vi "Filter Noise.vi"(8 "error in":errorcluster caption="error out") -> (0 "error out":errorcluster caption="error in")   [LabVIEW 2015, in "Debug.lvlib"]
uses:
  Debug.lvlib
  Support/Filter Noise State.ctl
  Sub VIs/DAQ/DAQ.lvlib
  Sub VIs/Utility VIs/Utility VIs.lvlib
  Sub VIs/Digital Signal Processing/Digital Signal Processing.lvlib
panel:
  out "进度条":u8(slide) scale=0.0..100.0
  out "DSP":dbl[](graph)
  out "Original Signal":dbl[](graph)
  in  "DOUT":bool
  in  "计算":bool
  in  "采集":bool
  out "状态栏":string
  in  "停止按钮":bool
  # "Filter Noise"
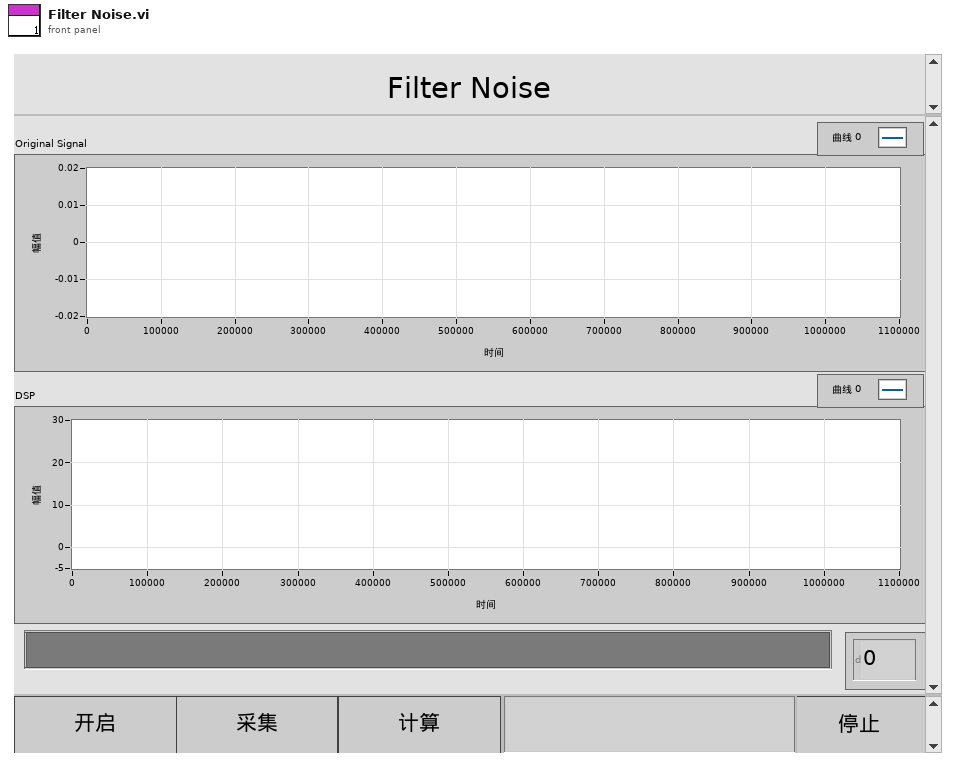
[diagram p1: front panel]
types:
  T1 = typedef "Debug.lvlib/Filter Noise State.ctl" = enum16{"Initialize", "Update Settings", "DOUT", "Sample", "Calculate", "Wait For Event", "Exit"}
  T2 = typedef "DAQ.lvlib/DAQ Configuration.ctl" = cluster{"hDevice":i32, "DevNum":u8, "Configuration Parameter":i32[], "READ_MAX_LEN":i32, "DO":bool[]}
  T3 = typedef "Digital Signal Processing.lvlib/DSP Configuration.ctl" = cluster{"Sampling Frequency":dbl, "filter type":T4, "RF Filter Low Frequency":dbl, "RF Filter High Frequency":dbl, "RF Filter Taps":i32, "window":T5, "RF window parameter":dbl, "filter type 2":T4, "Demodulated Filter Low Frequency":dbl, "Demodulated Filter HighFrequency":dbl, "Demodulated Filter Order":i32, "SPAN":i32, "Logarithmic Base":dbl, "Noise path":string, "Work position parameter":i32[]}
  T4 = typedef "NI_AALBase.lvlib/Filter Passband Type.ctl" = enum32{"Lowpass", "Highpass", "Bandpass", "Bandstop"}
  T5 = typedef "NI_AALPro.lvlib/windowTd.ctl" = u32
  T6 = typedef "Digital Signal Processing.lvlib/DSP Parameter.ctl" = cluster{"RF":cluster{"filter structure":enum32{"IIR 2nd Order", "IIR 4th Order"}, "Reverse Coefficients":dbl[], "Forward Coefficients":dbl[]}, "IIR Filter Cluster":cluster{"filter structure":enum32{"IIR 2nd Order", "IIR 4th Order"}, "Reverse Coefficients":dbl[], "Forward Coefficients":dbl[]}, "Noise Signal":dbl[], "SPAN":i32, "Logarithmic Base":dbl}
  T7 = cluster{"filter structure":enum32{"IIR 2nd Order", "IIR 4th Order"}, "Reverse Coefficients":dbl[], "Forward Coefficients":dbl[]}
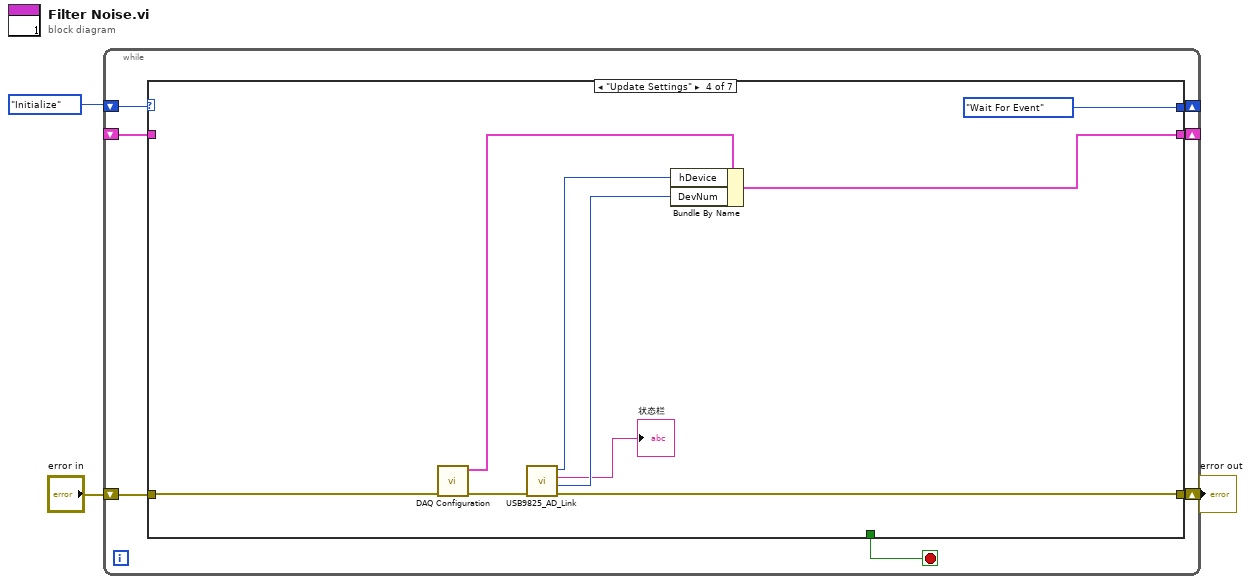
[diagram p0: block diagram]
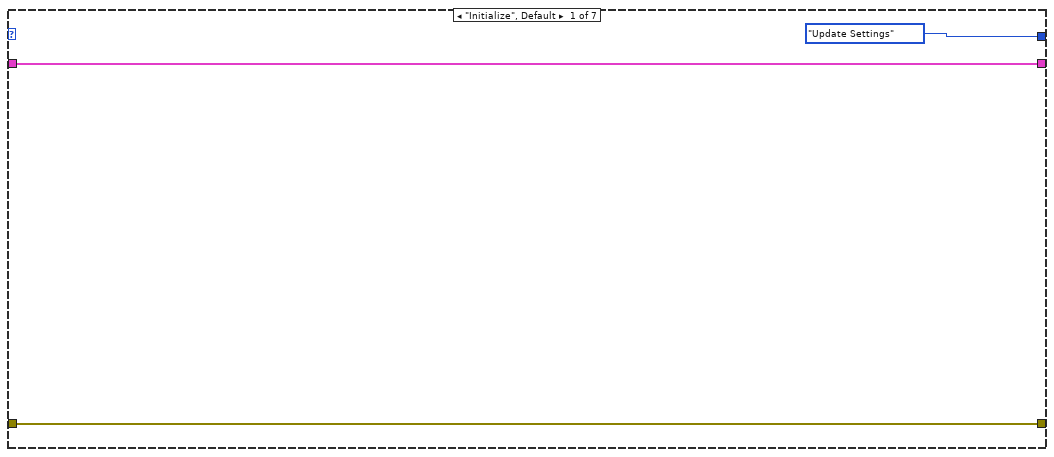
[diagram p2: hidden frame]
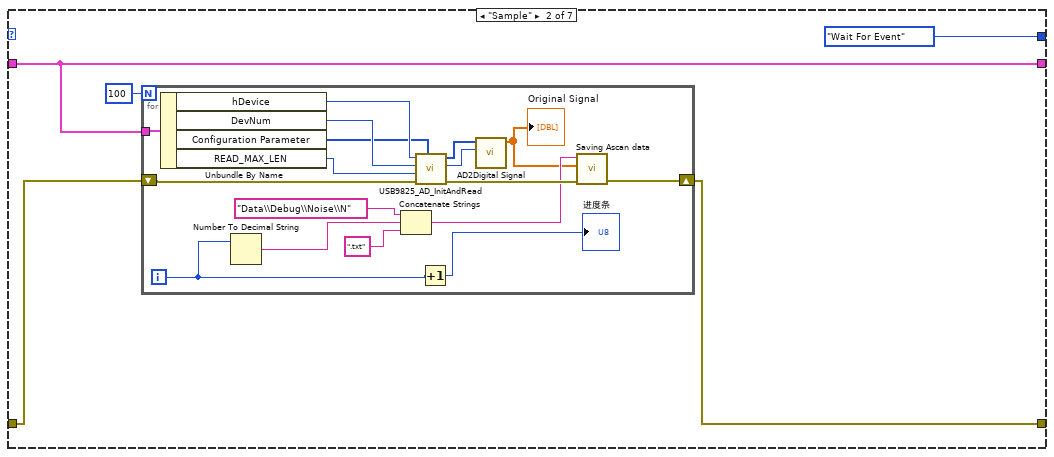
[diagram p3: hidden frame]
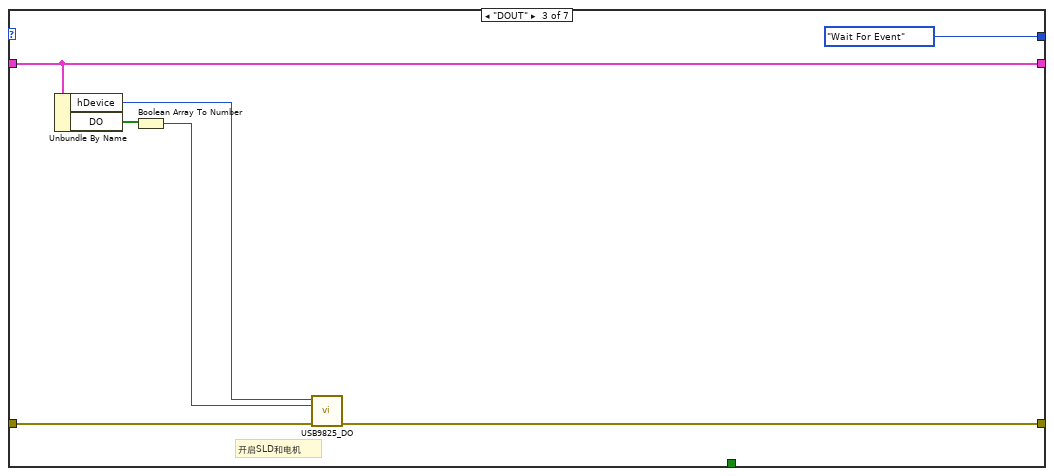
[diagram p4: hidden frame]
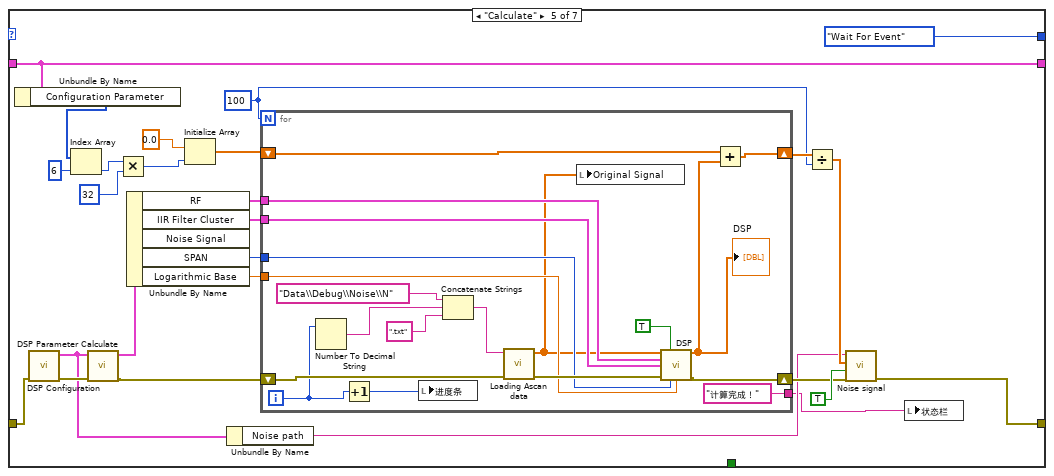
[diagram p5: hidden frame]
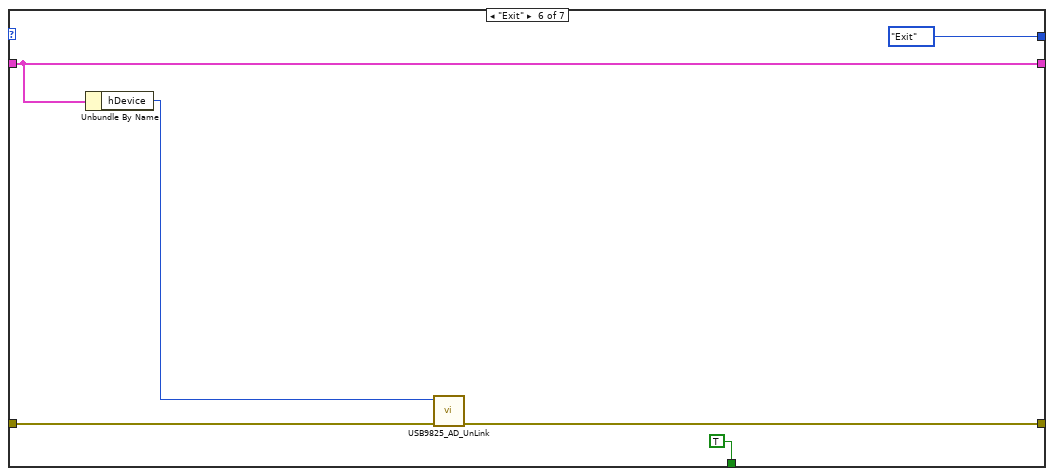
[diagram p6: hidden frame]
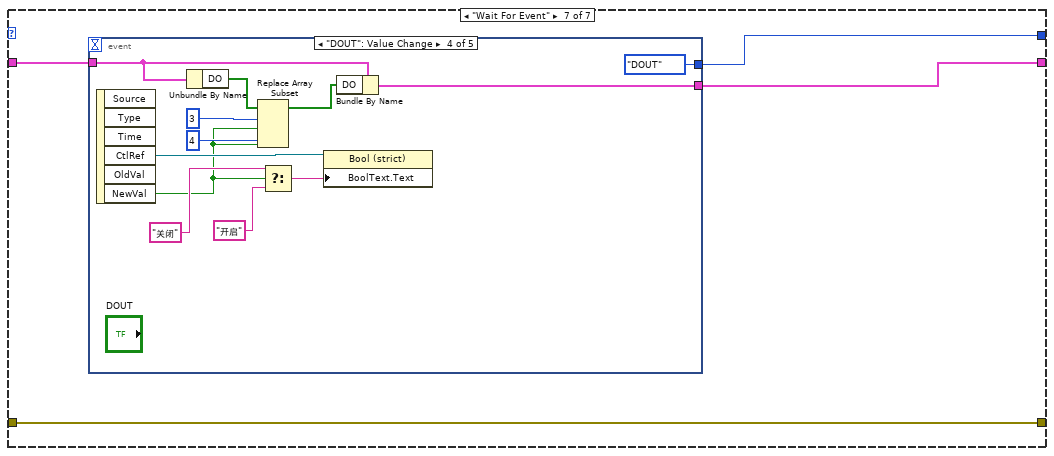
[diagram p7: hidden frame]
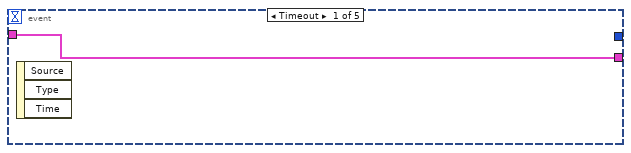
[diagram p8: hidden frame]
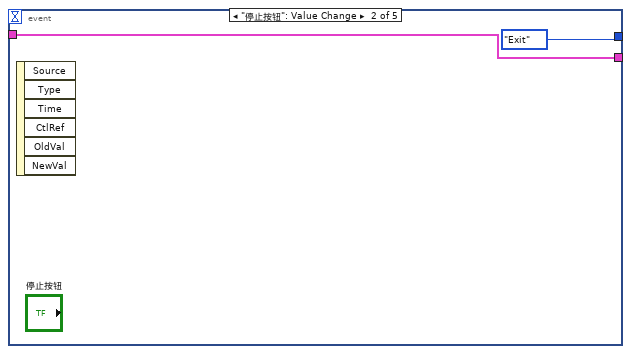
[diagram p9: hidden frame]
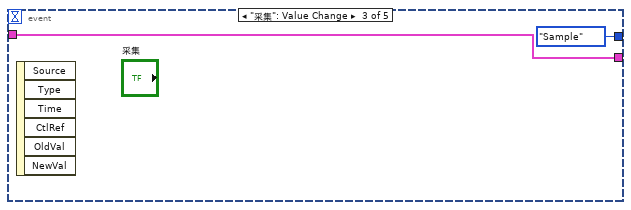
[diagram p10: hidden frame]
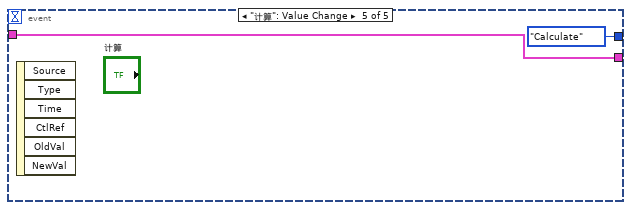
[diagram p11: hidden frame]
diagram:
  n1 = while {
    shift-right: [w9] -> _
    shift-left: Filter_Noise_State."Initialize" ("Calculation Distance State") -> [w10]
    shift-right: [w7] -> w2
    shift-left: "error in" -> [w6]
    shift-right: [w5] -> _
    shift-left: _ -> [w4]
    stop <- w8 stop-if-true
    n2 = case shown="\"Update Settings\"" w10 {
      tunnel: [Filter_Noise_State."Update Settings" ("Calculation Distance State") Filter_Noise_State."Wait For Event" ("Calculation Distance State") Filter_Noise_State."Wait For Event" ("Calculation Distance State") Filter_Noise_State."Wait For Event" ("Calculation Distance State") Filter_Noise_State."Wait For Event" ("Calculation Distance State") Filter_Noise_State."Exit" ("Calculation Distance State") w106] -> w9
      tunnel: [_ _ _ _ _ TRUE _] -> w8
      tunnel: w6 -> [w13 w17 w41 w50 w68 w100 w105]
      tunnel: [w13 w14 w40 w48 w53 w99 w105] -> w7
      tunnel: [w11 w15 w39 w44 w70 w98 w103] -> w5
      tunnel: w4 -> [w11 w15 w39 _ w70 w98 w104]
      frame "Initialize", Default {
      }
      frame "Sample" {
        n3 = for {
          N: 100 -> [_]
          tunnel: w15 -> [w35]
          shift-right: [w28] -> w14
          shift-left: w17 -> [w30]
          i -> [w20]
          n4 = Unbundle By Name(w35) -> ("hDevice"=w34:i32, "DevNum"=w33:u8, "Configuration Parameter"=w31:i32[], "READ_MAX_LEN"=w32:i32)
          n5 = Number To Decimal String(number=w20) -> (decimal integer string=w26:string)  [unwired: 1 in]
          n6 = Concatenate Strings("Data\\Debug\\Noise\\N" ("名称或相对路径"), w26, ".txt" ("字符串")) -> (w24:string)
          n7 = call "USB9825_AD_InitAndRead.vi"("Configuration Parameter"=w31, "错误输入（无错误）"=w30, "READ_MAX_LEN"=w32, "DevNum"=w33, "hDevice"=w34) -> ("错误输出"=w29:errorcluster, "通道数"=w22:i32, "AD"=w23:i16[])  [unwired: 3 in, 1 out]
          n8 = Increment(x=w20) -> (x+1=→"进度条":i32)
          n9 = call "AD2Digital Signal.vi"("通道数"=w22, "AD"=w23) -> ("CH1"=w21:dbl[])  [unwired: 8 in, 1 out]
          "Original Signal" <- w21
          n10 = call "Saving Ascan data.vi"("error in (no error)"=w29, "Ascan Data"=w21, "名称或相对路径"=w24) -> ("error out"=w28:errorcluster)  [unwired: 8 in]
        }
      }
      frame "DOUT" {
        # "开启SLD和电机"
        n11 = Unbundle By Name(w39) -> ("hDevice"=w38:i32, "DO"=w37:bool[])
        n12 = Boolean Array To Number(Boolean array=w37) -> (number=w36:u32)
        n13 = call "USB9825_DO.vi"("Error In"=w41, "pDO"=w36, "hDevice"=w38) -> ("Error Out"=w40:errorcluster)  [unwired: 8 in]
      }
      frame "Update Settings" {
        n14 = call "DAQ Configuration.vi"("error in (no error)"=w50) -> ("error out"=w49:errorcluster, "parameter output"=w47:T2)  [unwired: 9 in]
        n15 = call "USB9825_AD_Link.vi"("Error In"=w49) -> ("Error Out"=w48:errorcluster, "DevNum"=w45:i32, "设备属性"=→"状态栏":string, "hDevice"=w46:i32)  [unwired: 7 in]
        n16 = Bundle By Name(cluster=w47, "hDevice"=w46, "DevNum"=w45) -> (w44:T2)
      }
      frame "Calculate" {
        w59 = 100
        n17 = Unbundle By Name(w70) -> ("Configuration Parameter"=w69:i32[])
        n18 = call "DSP Configuration.vi"("error in (no error)"=w68) -> ("error out"=w67:errorcluster, "DSP Parameter Output"=w55:T3)  [unwired: 9 in]
        n19 = Index Array(array=w69, index=6 ("索引")) -> (element=w75:i32)
        n20 = call "DSP Parameter Calculate.vi"("error in (no error)"=w67, "DSP Configuration"=w55) -> ("error out"=w66:errorcluster, "DSP Parameter"=w65:T6)  [unwired: 8 in]
        n21 = Multiply(x=w75, y=32) -> (x*y=w73:i32)
        n22 = Unbundle By Name(w65) -> ("RF"=w64:T7, "IIR Filter Cluster"=w63:T7, "SPAN"=w62:i32, "Logarithmic Base"=w61:dbl)  [unwired: 1 out]
        n23 = Initialize Array(0.0 ("元素"), w73) -> (w71:dbl[])
        n24 = Unbundle By Name(w55) -> ("Noise path"=w54:string)
        n25 = for {
          N: w59 -> [_]
          shift-right: [w90] -> w57
          shift-left: w66 -> [w96]
          shift-right: [w89] -> w60
          shift-left: w71 -> [w88]
          tunnel: w64 -> [w87]
          tunnel: w63 -> [w86]
          tunnel: w62 -> [w85]
          tunnel: w61 -> [w84]
          tunnel: ["计算完成！"] -> w52
          i -> [w82]
          n26 = Number To Decimal String(number=w82) -> (decimal integer string=w94:string)  [unwired: 1 in]
          n27 = Increment(x=w82) -> (x+1=w81:i32)
          n28 = local write "进度条"(w81) -> ()
          n29 = Concatenate Strings("Data\\Debug\\Noise\\N" ("名称或相对路径"), w94, ".txt" ("字符串")) -> (w92:string)
          n30 = call "Loading Ascan data.vi"("error in (no error)"=w96, "名称或相对路径"=w92) -> ("error out"=w91:errorcluster, "first row"=w79:dbl[])  [unwired: 8 in]
          n31 = local write "Original Signal"(w79) -> ()
          n32 = call "DSP.vi"("Input Signal"=w79, "Smooth(F : Don't)"=TRUE, "RF"=w87, "IIR Filter Cluster"=w86, "error in (no error)"=w91, "SPAN"=w85, "Logarithmic Base"=w84) -> ("DSP signal"=w80:dbl[], "error out"=w90:errorcluster)  [unwired: 7 in]
          "DSP" <- w80
          n33 = Add(x=w88, y=w80) -> (x+y=w89:dbl[])
        }
        n34 = Divide(x=w60, y=w59) -> (x/y=w56:dbl[])
        n35 = call "Noise signal.vi"("错误输入"=w57, "写入（非为读取）"=TRUE, "input signal"=w56, "Path"=w54) -> ("错误输出"=w53:errorcluster)  [unwired: 6 in, 1 out]
        n36 = local write "状态栏"(w52) -> ()
      }
      frame "Exit" {
        n37 = Unbundle By Name(w98) -> ("hDevice"=w97:i32)
        n38 = call "USB9825_AD_UnLink.vi"("Error In"=w100, "hDevice"=w97) -> ("Error Out"=w99:errorcluster)  [unwired: 9 in]
      }
      frame "Wait For Event" {
        n39 = event shown="[3] \"DOUT\": Value Change" {
          selector: _ -> [_ _ _ _ _]
          dyn-events: _ -> [_ _ _ _ _]
          timeout: _ -> [_ _ _ _ _]
          tunnel: [_ Filter_Noise_State."Exit" ("Calculation Distance State") Filter_Noise_State."Sample" ("Calculation Distance State") Filter_Noise_State."DOUT" ("Calculation Distance State") Filter_Noise_State."Calculate" ("Calculation Distance State")] -> w106
          tunnel: w104 -> [w107 w108 w110 w114 w124]
          tunnel: [w107 w108 w110 w112 w124] -> w103
          event Timeout {
            n40 = event-data() -> ()  [unwired: 1 in, 3 out]
          }
          event "停止按钮": Value Change {
            n41 = event-data() -> ()  [unwired: 1 in, 6 out]
          }
          event "采集": Value Change {
            n42 = event-data() -> ()  [unwired: 1 in, 6 out]
          }
          event "DOUT": Value Change {
            n43 = event-data() -> ("CtlRef"=w122:refnum<vi>, "NewVal"=w115:bool)  [unwired: 1 in, 4 out]
            n44 = Unbundle By Name(w114) -> ("DO"=w118:bool[])
            n45 = Replace Array Subset(array=w118, new element #1=w115, index #1=3 ("索引"), new element #2=w115, index #2=4 ("索引")) -> (w113:bool[])
            n46 = Select(t="关闭", s=w115, f="开启") -> (s? t:f=w121:string)
            n47 = property class="Bool (strict)"(reference=w122, "BoolText.Text"=w121) -> ()  [unwired: 1 in, 2 out]
            n48 = Bundle By Name(cluster=w114, "DO"=w113) -> (w112:T2)
          }
          event "计算": Value Change {
            n49 = event-data() -> ()  [unwired: 1 in, 6 out]
          }
        }
      }
    }
  }
  "error out" <- w2
